vi "Sort data sheet.vi"(8 "error in":errorcluster, 10 "Config File Test Number":string[](array[string]), 11 "Input Data Sheet":string[][](array[string])) -> (0 "error out":errorcluster, 3 "Output Data Sheet":string[][](array[string]))   [LabVIEW 2020, in "GUCalibration2.lvlib"]
uses:
  GUCalibration2.lvlib
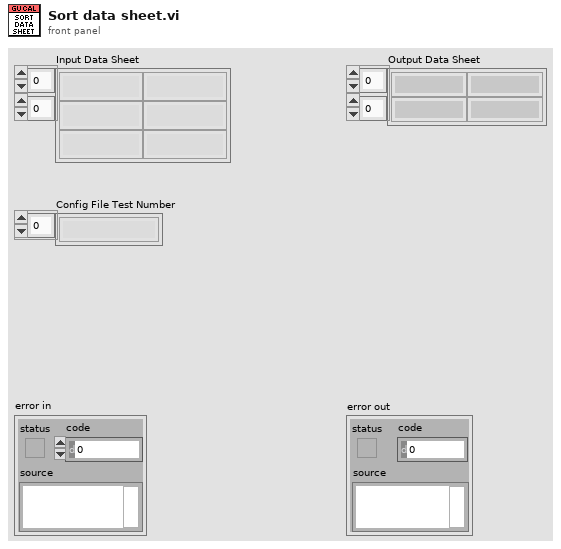
[diagram p1: front panel]
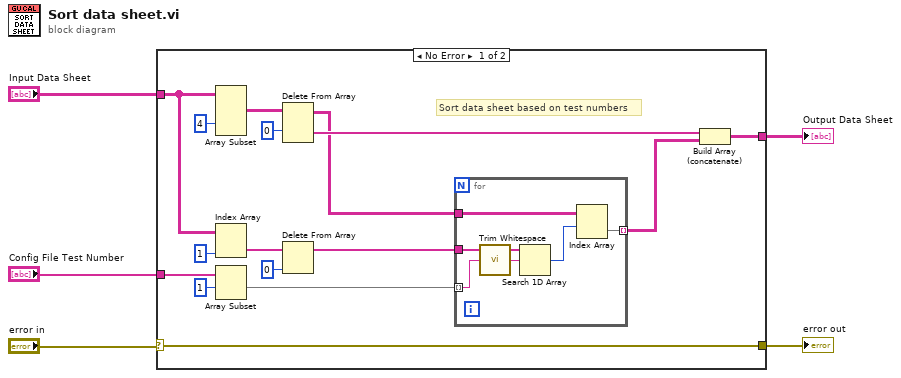
[diagram p0: block diagram]
diagram:
  n1 = case shown="No Error" "error in" {
    selector: "error in" -> [w18 w28]
    tunnel: "Input Data Sheet" -> [w10 _]
    tunnel: [w19 _] -> w4
    tunnel: "Config File Test Number" -> [w7 _]
    tunnel: [w18 w28] -> w2
    frame No Error {
      # "Sort data sheet based on test numbers"
      n2 = Array Subset(array=w10, index (col)=4 ("disabled index (col)")) -> (w21:string[][])  [unwired: 3 in]
      n3 = Index Array(array=w10, index (col)=1 ("disabled index (col)")) -> (element=w12:string[])  [unwired: 1 in]
      n4 = Array Subset(array=w7, index=1) -> (w8:string[])  [unwired: 1 in]
      n5 = Delete From Array(array=w21, index (row)=0) -> (deleted portion=w16:string[], array with subset deleted=w14:string[][])  [unwired: 2 in]
      n6 = Delete From Array(array=w12, index=0) -> (array with subset deleted=w9:string[])  [unwired: 1 in, 1 out]
      n7 = for {
        tunnel: w8 -> [w26] mode=indexing
        tunnel: w14 -> [w24]
        tunnel: w9 -> [w27]
        tunnel: [w23] -> w20 mode=indexing
        n8 = call <vilib>:"Trim Whitespace.vi"("string"=w26) -> ("trimmed string"=w22:string)  [unwired: 1 in]
        n9 = Search 1D Array(1D array=w27, element=w22) -> (index of element=w25:i32)  [unwired: 1 in]
        n10 = Index Array(array=w24, index (row)=w25) -> (element=w23:string[])  [unwired: 1 in]
      }
      n11 = Build Array (concatenate)(w16, w20) -> (w19:string[][])
    }
    frame Error {
    }
  }
  "Output Data Sheet" <- w4
  "error out" <- w2
